vi "Avg Temp Array Fix.vi"(11 "Input Array":dbl[][][](array[numeric])) -> (3 "Output Array":dbl[][][](array[numeric]))   [LabVIEW 2017]
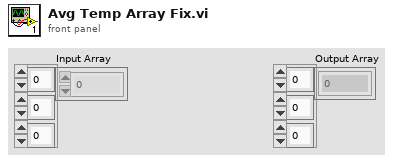
[diagram p1: front panel]
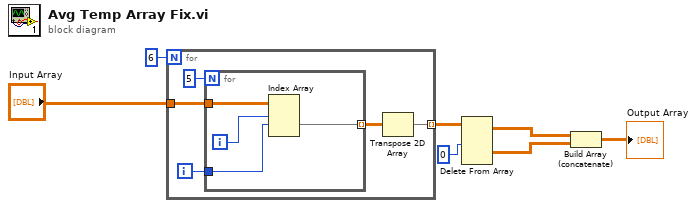
[diagram p0: block diagram]
diagram:
  n1 = for {
    N: 6 -> [_]
    tunnel: "Input Array" -> [w11]
    tunnel: [w8] -> w3 mode=indexing
    i -> [w10]
    n2 = for {
      N: 5 -> [_]
      tunnel: w11 -> [w15]
      tunnel: w10 -> [w14]
      tunnel: [w13] -> w9 mode=indexing
      i -> [w16]
      n3 = Index Array(array=w15, index (dim 0)=w16, index (dim 1)=w14) -> (element=w13:dbl[])  [unwired: 1 in]
    }
    n4 = Transpose 2D Array(2D array=w9) -> (transposed array=w8:dbl[][])
  }
  n5 = Delete From Array(array=w3, index (dim 0)=0 ("index (page)")) -> (deleted portion=w4:dbl[][], array with subset deleted=w2:dbl[][][])  [unwired: 3 in]
  n6 = Build Array (concatenate)(w2, w4) -> (→"Output Array":dbl[][][])
